vi "Create_filter_points.vi"(1 "Non-Blank Rows":bool[](array[boolean]), 5 "Precision":string, 6 "Channel to Filter On":i32, 7 "Tolerance":dbl=1.0 format="%.2f", 8 "Index":i32, 9 "Filter Bins 1":i32[](array[numeric]), 10 "Ch Values In":string[][](array[string])) -> (0 "Unchanged?":bool, 2 "Accept array":bool[][](array[boolean]), 3 "Filter Bins Out":i32[](array[numeric]), 4 "Bin Names":string[](array[string]))   [LabVIEW 2014]
uses:
  Results_plotter_Global.vi
panel:
  in  "Filter Info":T1={"Filter Bins"=[], "Channel to Filter On"=0, "Bin Matches"=[], "Number of Rows"=0, "Bin Names"=[], "Tolerance"=1.0, "Indicies for all bins"=[]} {"Tolerance" format="%.2f"}
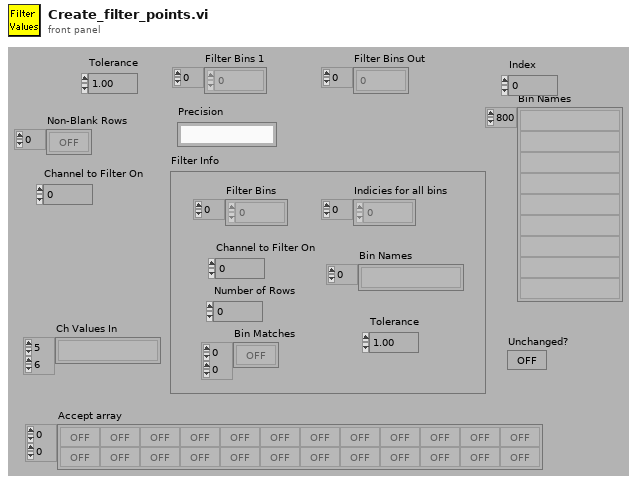
[diagram p1: front panel]
types:
  T1 = cluster{"Filter Bins":i32[], "Channel to Filter On":i32, "Bin Matches":bool[][], "Number of Rows":i32, "Bin Names":string[], "Tolerance":dbl, "Indicies for all bins":i32[]}
  T2 = cluster{"Filter Bins":i32[], "Channel to Filter On":i32, "Bin Matches":bool[][], "Number of Rows":i32, "Bin Names":string[], "Tolerance":dbl, "Indicies for all bins":i32[]}[]
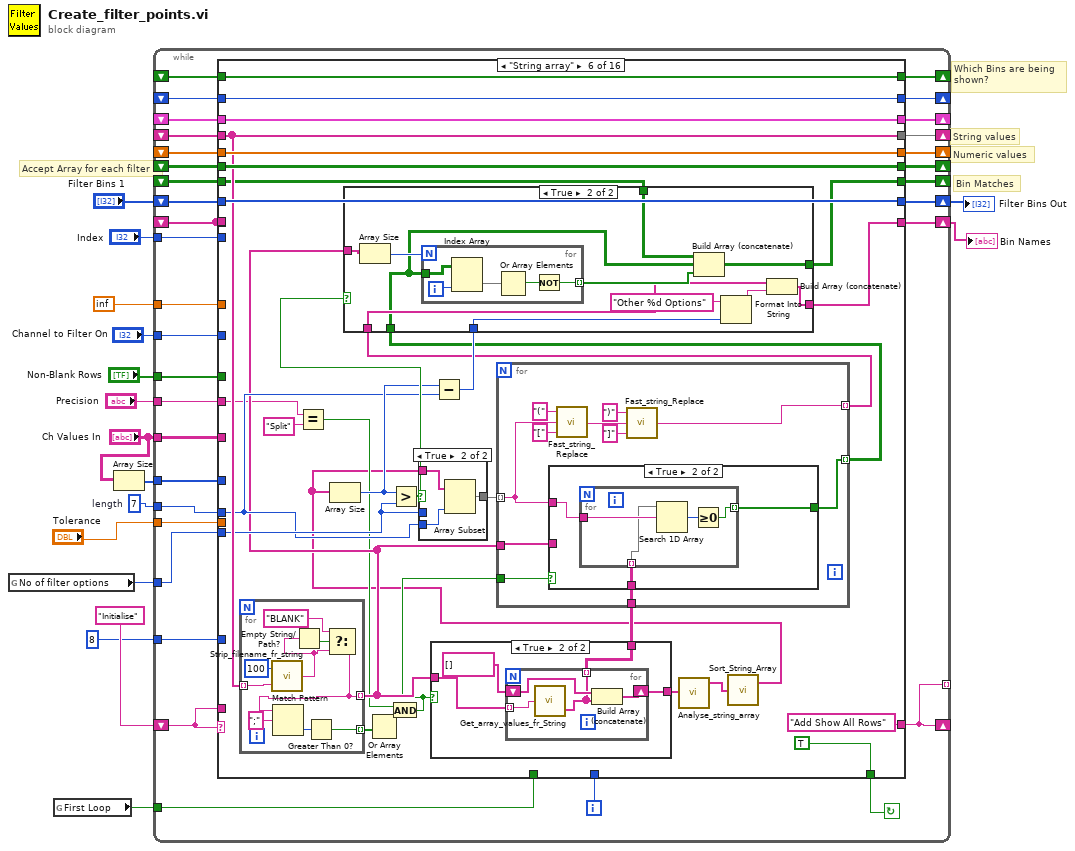
[diagram p0: block diagram]
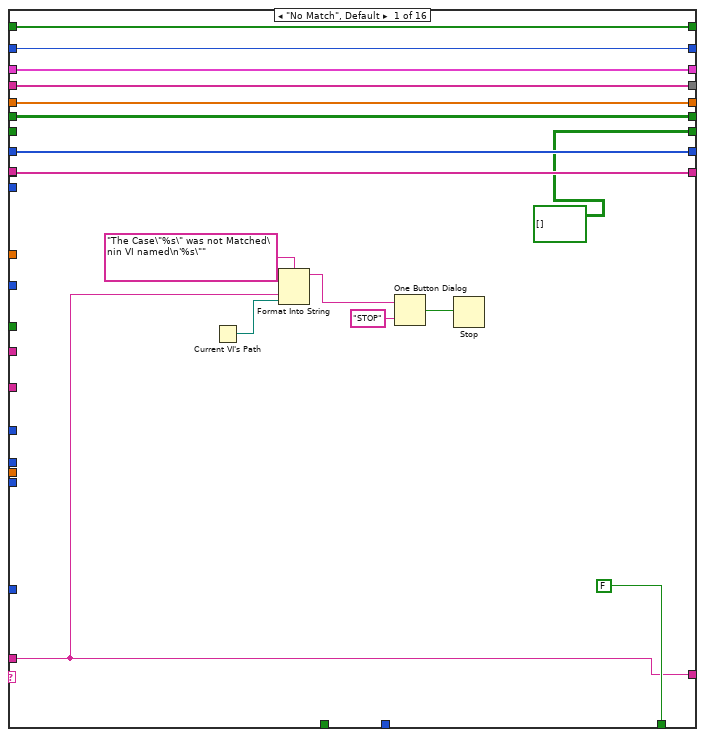
[diagram p2: hidden frame]
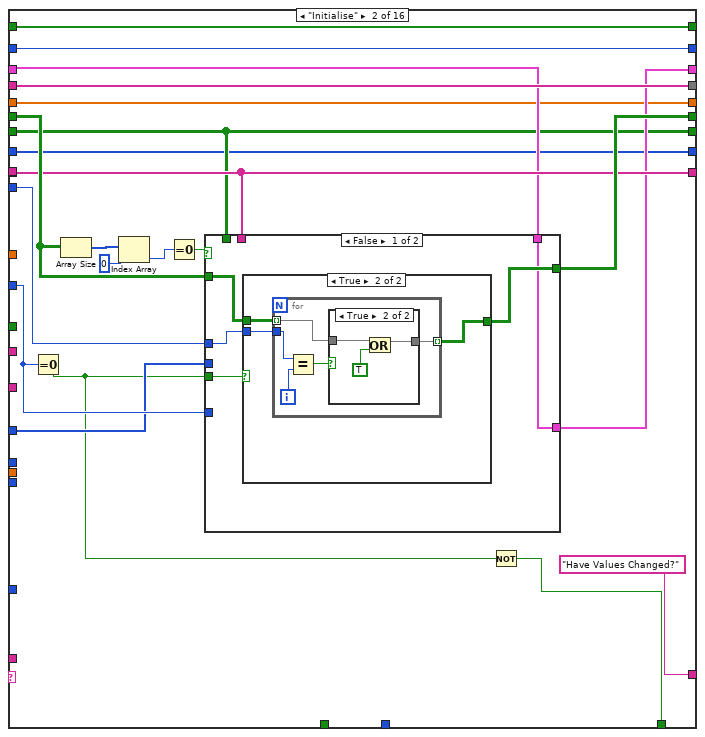
[diagram p3: hidden frame]
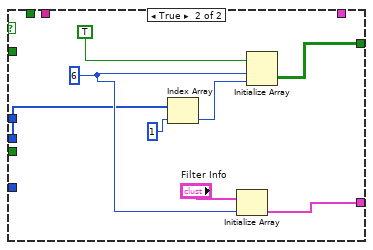
[diagram p6: hidden frame]
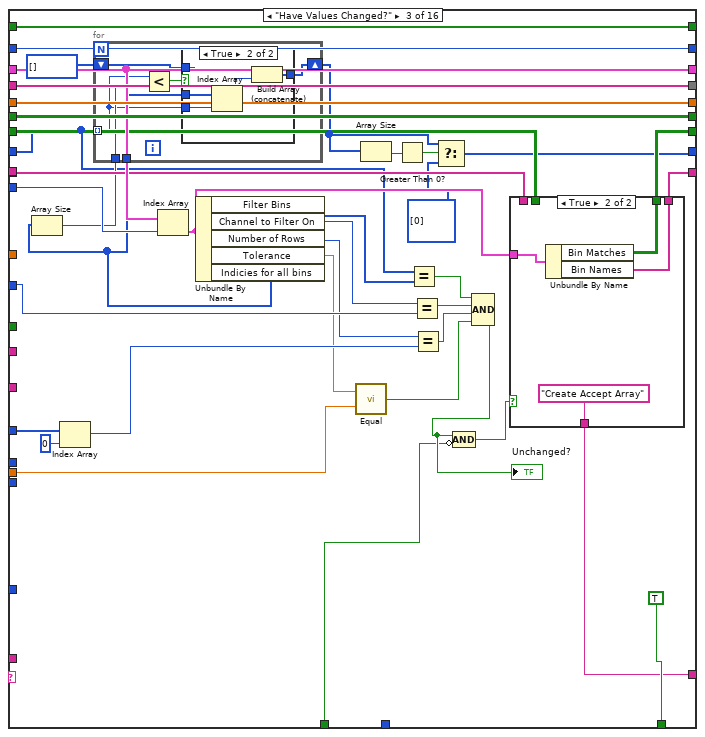
[diagram p7: hidden frame]
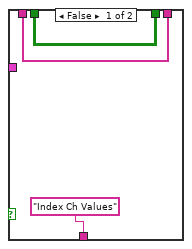
[diagram p9: hidden frame]
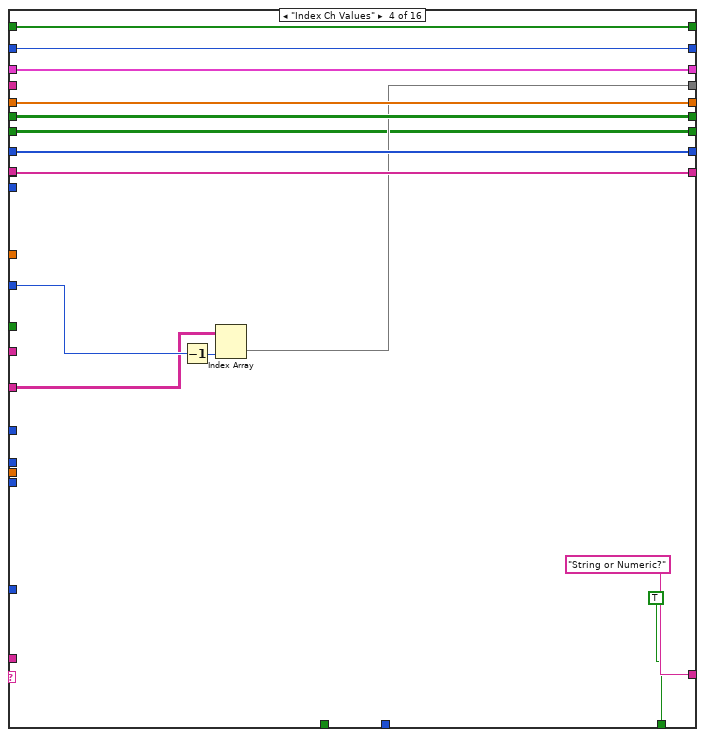
[diagram p10: hidden frame]
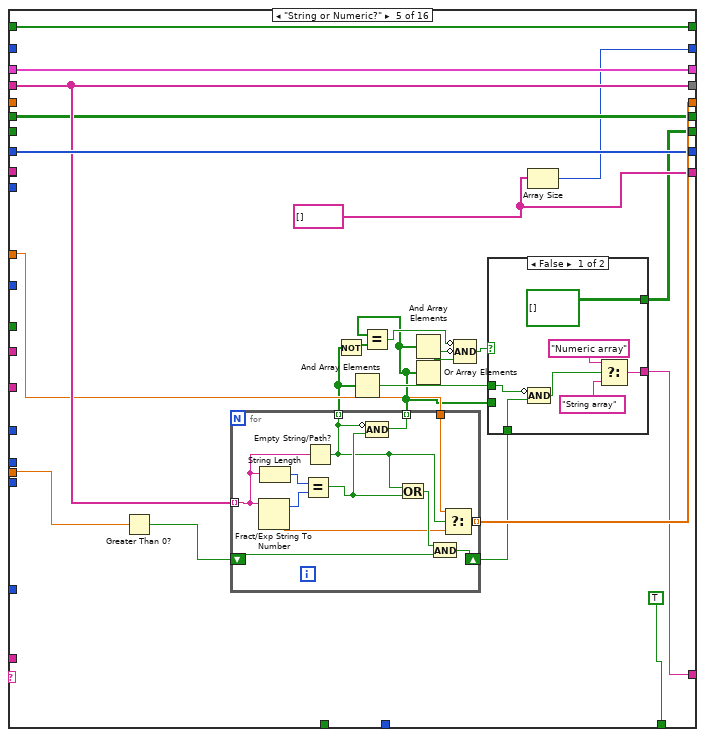
[diagram p11: hidden frame]
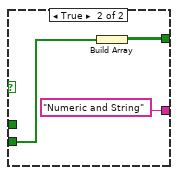
[diagram p12: hidden frame]
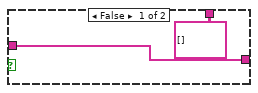
[diagram p13: hidden frame]
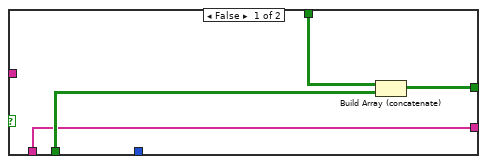
[diagram p14: hidden frame]
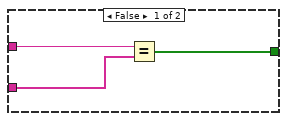
[diagram p16: hidden frame]
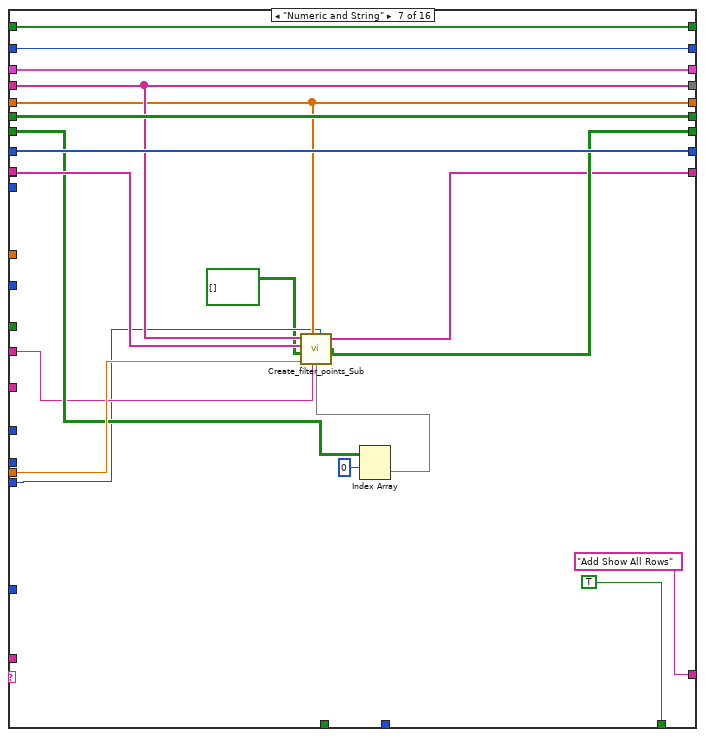
[diagram p17: hidden frame]
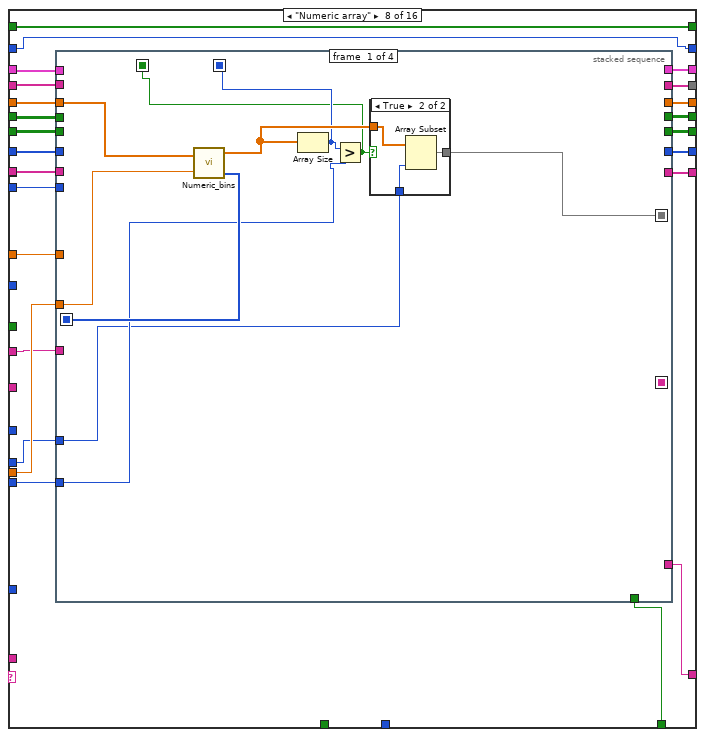
[diagram p18: hidden frame]
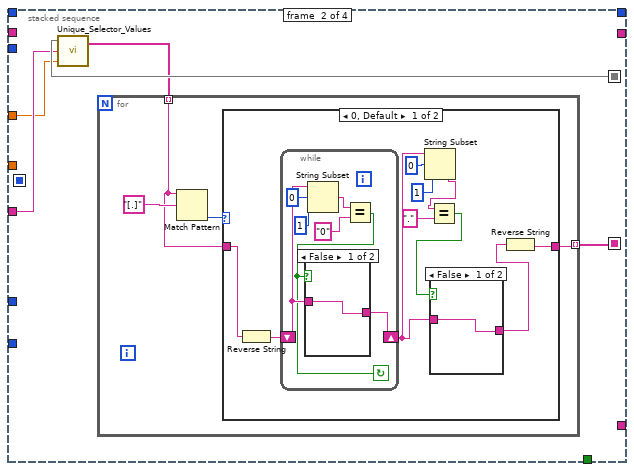
[diagram p20: hidden frame]
diagram:
  w5 = 7  # length
  # "Which Bins are being\nshown?"
  # "Accept Array for each filter"
  # "String values"
  # "Bin Matches"
  # "Numeric values"
  n1 = global read "Results_plotter_Global.vi" "No of filter options"() -> (w6:i32)
  n2 = global read "Results_plotter_Global.vi" "First Loop"() -> (w9:bool)
  n3 = Array Size(array="Ch Values In") -> (size(s)=w11:i32[])
  n4 = while {
    tunnel: "Non-Blank Rows" -> [w30]
    tunnel: w11 -> [w32]
    tunnel: "Channel to Filter On" -> [w34]
    shift-left: _ -> [w36]
    shift-right: [w35] -> _
    shift-left: _ -> [w37]
    shift-right: [w33] -> _
    shift-left: "Filter Bins 1" -> [w39]
    shift-right: [w38] -> w3
    tunnel: "Index" -> [w41]
    shift-left: _ -> [w40]
    shift-right: [w42] -> w14
    shift-left: _ -> [w27]
    shift-right: [w24] -> _
    shift-left: _ -> [w46]
    shift-right: [w45] -> _
    shift-left: _ -> [w43]
    shift-right: [w48] -> _
    shift-left: "Initialise" -> [w44]
    shift-right: [w17] -> _
    tunnel: inf -> [w49]
    tunnel: "Ch Values In" -> [w50]
    tunnel: w9 -> [w29]
    tunnel: "Tolerance" -> [w28]
    shift-right: [w26] -> _
    shift-left: _ -> [w25]
    tunnel: "Precision" -> [w23]
    shift-right: [w22] -> _
    shift-left: _ -> [w21]
    tunnel: w6 -> [w20]
    tunnel: w5 -> [w19]
    tunnel: 8 ("y") -> [w18]
    tunnel: [w17] -> _ mode=indexing
    i -> [w31]
    stop <- w47 continue-if-true
    n5 = case shown="\"String array\"" w44 {
      tunnel: w50 -> [_ _ _ w175 _ _ _ _ _ _ _ _ _ _ _ _]
      tunnel: w49 -> [_ _ _ _ w201 _ _ w358 _ _ _ _ _ _ _ _]
      tunnel: [w65 w73 w151 w183 w208 w260 w332 w365 w482 w500 w520 w562 w614 w632 w659 w698] -> w48
      tunnel: [w55 "Have Values Changed?" w135 "String or Numeric?" w192 "Add Show All Rows" "Add Show All Rows" w367 w465 "Create Accept Array" "Add Number of hits" "Relocate Selector?" w603 "Stop invalid selections" "Update shift Register" "End"] -> w17
      tunnel: [FALSE w76 TRUE TRUE TRUE TRUE TRUE w368 TRUE TRUE TRUE TRUE TRUE TRUE TRUE FALSE] -> w47
      tunnel: w46 -> [w64 w83 w150 w182 w202 w257 w341 w363 w481 w499 w515 w559 w612 w631 w658 w697]
      tunnel: [w64 w84 w150 w182 w202 w257 w341 w362 w481 w499 w514 w559 w612 w631 w658 w697] -> w45
      tunnel: w44 -> [w55 _ _ _ _ _ _ _ _ _ _ _ _ _ _ _]
      tunnel: w43 -> [w65 w73 w151 w183 _ w260 w332 w364 w482 w500 w520 w562 w614 w632 w659 w698]
      tunnel: [w63 w79 w134 w180 w188 w247 w333 w366 w469 w487 w518 w557 w611 w629 w656 w677] -> w42
      tunnel: w41 -> [_ w82 w148 _ _ _ _ w357 _ _ w517 w563 w601 w628 _ w695]
      tunnel: w27 -> [_ w74 w136 w174 _ w250 w335 w360 w475 w492 w507 w551 w613 w624 w654 w688]
      tunnel: w40 -> [w63 w79 w133 w180 _ _ w336 w351 w474 w488 w518 w554 w611 w629 w656 w680]
      tunnel: w40 -> [_ _ _ _ _ _ _ _ _ _ _ _ _ _ _ _]
      tunnel: w39 -> [w54 w72 w114 w181 w206 w256 w340 w359 w485 w503 w512 w566 w616 w622 w652 w675]
      tunnel: [w54 w72 w115 w181 w206 w256 w340 w352 w485 w503 w512 w566 w616 w617 w648 w674] -> w38
      tunnel: w37 -> [w62 w81 w149 _ w204 w254 w339 w356 w483 w501 w521 w564 w615 w630 w657 w696]
      tunnel: w36 -> [w61 w77 w147 w179 w205 w258 w342 w354 w484 w502 w522 w565 w609 w620 w651 w694]
      tunnel: [w61 w78 w147 w179 w205 w258 w342 w353 w484 w502 w522 w565 w609 w620 w651 w693] -> w35
      tunnel: w34 -> [_ w80 w146 w177 _ _ _ _ _ _ _ _ _ _ _ w687]
      tunnel: [w62 w81 w149 w176 w204 w254 w339 w355 w483 w501 w521 w564 w615 w630 w657 w696] -> w33
      tunnel: [bool[][] [] w74 w123 w174 w187 w248 w334 w361 w464 w491 w507 w551 w613 w624 w654 w688] -> w24
      tunnel: w32 -> [_ w71 w145 _ _ _ _ _ w479 _ _ _ _ _ _ w692]
      tunnel: w31 -> [_ _ _ _ _ _ _ _ _ _ _ _ _ _ _ _]
      tunnel: w30 -> [_ _ _ _ _ _ _ _ _ _ w511 w561 _ _ _ _]
      tunnel: w29 -> [_ _ w127 _ _ _ _ _ _ _ _ _ _ _ _ _]
      tunnel: w28 -> [_ _ w126 _ w191 _ w338 w350 _ _ _ _ _ _ _ w683]
      tunnel: [w53 w68 w125 w173 w190 w255 w331 w345 w471 w496 w509 w558 w600 w619 w650 w682] -> w26
      tunnel: w25 -> [w53 w68 w125 w173 _ w255 w331 w345 w471 w496 w509 w558 w600 w619 w650 w682]
      tunnel: w23 -> [_ _ _ _ _ w236 w330 w349 _ _ _ _ _ _ _ _]
      tunnel: [w51 w67 w124 w172 w189 w253 w329 w348 w470 w486 w508 w556 w599 w618 w649 w681] -> w22
      tunnel: w21 -> [w51 w67 w124 w172 w189 w253 w329 w348 w470 w486 w508 _ w599 w618 w649 w681]
      tunnel: w20 -> [_ _ _ _ _ w251 w328 w347 _ _ _ w543 _ _ _ _]
      tunnel: w19 -> [_ _ _ _ _ w245 _ w346 _ _ _ _ _ _ _ _]
      tunnel: w18 -> [_ _ _ _ _ _ _ _ w462 _ _ w545 _ _ _ _]
      frame "No Match", Default {
        n6 = Current VI's Path() -> (path=w56:path)
        n7 = Format Into String(format string="The Case\"%s\" was not Matched\nin VI named\n'%s\"" ("Format String"), w55, w56) -> (resulting string=w59:string)  [unwired: 2 in, 1 out]
        n8 = One Button Dialog(message=w59, button name ("OK")="STOP") -> (true=w57:bool)
        n9 = Stop(stop? (T)=w57) -> ()
      }
      frame "Initialise" {
        n10 = Equal To 0?(x=w80) -> (x = 0?=w70:bool)
        n11 = Array Size(array=w83) -> (size(s)=w87:i32[])
        n12 = Index Array(array=w87, index=0 ("Index")) -> (element=w85:i32)
        n13 = Equal To 0?(x=w85) -> (x = 0?=w69:bool)
        n14 = case shown="False" w69 {
          tunnel: [w92 w112] -> w84
          tunnel: w83 -> [w91 _]
          tunnel: w82 -> [w90 _]
          tunnel: w70 -> [w89 _]
          tunnel: w80 -> [_ _]
          tunnel: w79 -> [_ _]
          tunnel: [w88 w110] -> w78
          tunnel: w77 -> [w88 _]
          tunnel: w74 -> [_ _]
          tunnel: w71 -> [_ w107]
          frame False {
            n15 = case shown="True" w89 {
              tunnel: [w93 w95] -> w92
              tunnel: w91 -> [w93 w94]
              tunnel: w90 -> [_ w96]
              frame False {
              }
              frame True {
                n16 = for {
                  tunnel: w96 -> [w101]
                  tunnel: [w98] -> w95 mode=indexing
                  tunnel: w94 -> [w97] mode=indexing
                  i -> [w100]
                  n17 = Equal?(x=w101, y=w100) -> (x = y?=w99:bool)
                  n18 = case shown="True" w99 {
                    tunnel: [w102 w103] -> w98
                    tunnel: w97 -> [w102 w104]
                    frame False {
                    }
                    frame True {
                      n19 = Or(x=w104, y=TRUE) -> (x .or. y?=w103:bool[])
                    }
                  }
                }
              }
            }
          }
          frame True {
            w111 = 6 ("Dimension Size")
            n20 = Index Array(array=w107, index=1 ("Index")) -> (element=w108:i32)
            n21 = Initialize Array("Filter Info", w111) -> (w110:T2)
            n22 = Initialize Array(TRUE, w111, w108) -> (w112:bool[][])
          }
        }
        n23 = Not(x=w70) -> (.not. x?=w76:bool)
      }
      frame "Have Values Changed?" {
        n24 = Index Array(array=w145, index=0 ("Index")) -> (element=w141:i32)
        n25 = Index Array(array=w147, index=w148) -> (element=w137:T1)
        n26 = Unbundle By Name(w137) -> ("Filter Bins"=w132:i32[], "Channel to Filter On"=w143:i32, "Number of Rows"=w142:i32, "Tolerance"=w129:dbl, "Indicies for all bins"=w122:i32[])
        n27 = Array Size(array=w122) -> (size(s)=w121:i32)
        n28 = for {
          tunnel: w114 -> [w156] mode=indexing
          tunnel: w122 -> [w158]
          tunnel: w121 -> [w157]
          shift-right: [w154] -> w117
          shift-left: i32[] [] -> [w153]
          n29 = Less?(x=w156, y=w157) -> (x < y?=w155:bool)
          n30 = case shown="True" w155 {
            tunnel: w158 -> [_ w164]
            tunnel: w156 -> [_ w163]
            tunnel: [w159 w161] -> w154
            tunnel: w153 -> [w159 w160]
            frame False {
            }
            frame True {
              n31 = Index Array(array=w164, index=w163) -> (element=w162:i32)
              n32 = Build Array (concatenate)(w160, w162) -> (w161:i32[])
            }
          }
        }
        n33 = call "Equal.vi"("Input2"=w126, "Input1"=w129) -> ("Equal?"=w128:bool)
        n34 = Array Size(array=w117) -> (size(s)=w119:i32)
        n35 = Greater Than 0?(x=w119) -> (x > 0?=w118:bool)
        n36 = Equal?(x=w114, y=w132) -> (x = y?=w140:bool)
        n37 = Equal?(x=w143, y=w146) -> (x = y?=w139:bool)
        n38 = Equal?(x=w142, y=w141) -> (x = y?=w138:bool)
        n39 = Select(t=w117, s=w118, f=i32[] [0]) -> (s? t:f=w115:i32[])
        n40 = Compound Arithmetic op=AND(w140, w139, w138, w128) -> (w130:bool)
        "Unchanged?" <- w130
        n41 = Compound Arithmetic op=AND(w130, invert w127) -> (w131:bool)
        n42 = case shown="True" w131 {
          tunnel: w137 -> [_ w171]
          tunnel: [w165 w169] -> w123
          tunnel: w136 -> [w165 _]
          tunnel: ["Index Ch Values" "Create Accept Array"] -> w135
          tunnel: [w166 w170] -> w134
          tunnel: w133 -> [w166 _]
          frame False {
          }
          frame True {
            n43 = Unbundle By Name(w171) -> ("Bin Matches"=w169:bool[][], "Bin Names"=w170:string[])
          }
        }
      }
      frame "Index Ch Values" {
        n44 = Decrement(x=w177) -> (x-1=w178:i32)
        n45 = Index Array(array=w175, index (col)=w178) -> (element=w176:string[])  [unwired: 1 in]
      }
      frame "String or Numeric?" {
        w188 = string[] []
        n46 = Greater Than 0?(x=w191) -> (x > 0?=w207:bool)
        n47 = for {
          tunnel: w204 -> [w223] mode=indexing
          shift-right: [w228] -> w193
          shift-left: w207 -> [w229]
          tunnel: [w227] -> w208 mode=indexing
          tunnel: [w221] -> w196 mode=indexing
          tunnel: w201 -> [w220]
          tunnel: [w219] -> w186 mode=indexing
          n48 = Fract/Exp String To Number(string=w223) -> (offset past number=w225:i32, number=w226:dbl)  [unwired: 3 out]
          n49 = String Length(string=w223) -> (length=w224:i32)
          n50 = Equal?(x=w224, y=w225) -> (x = y?=w222:bool)
          n51 = Empty String/Path?(string/path=w223) -> (empty?=w221:bool)
          n52 = Compound Arithmetic op=AND(invert w221, w222) -> (w219:bool)
          n53 = Or(x=w221, y=w222) -> (x .or. y?=w230:bool)
          n54 = And(x=w230, y=w229) -> (x .and. y?=w228:bool)
          n55 = Select(t=w220, s=w221, f=w226) -> (s? t:f=w227:dbl)
        }
        n56 = Not(x=w196) -> (.not. x?=w195:bool[])
        n57 = And Array Elements(Boolean array=w196) -> (logical AND=w194:bool)
        n58 = Equal?(x=w186, y=w195) -> (x = y?=w197:bool)
        n59 = And Array Elements(Boolean array=w186) -> (logical AND=w200:bool)
        n60 = Or Array Elements(Boolean array=w186) -> (logical OR=w199:bool)
        n61 = Compound Arithmetic op=AND(invert w197, invert w200, w199) -> (w198:bool)
        n62 = case shown="False" w198 {
          tunnel: w194 -> [w215 _]
          tunnel: w193 -> [w214 _]
          tunnel: [w210 "Numeric and String"] -> w192
          tunnel: [bool[][] [] w216] -> w187
          tunnel: w186 -> [_ w217]
          frame False {
            n63 = Compound Arithmetic op=AND(invert w215, w214) -> (w211:bool)
            n64 = Select(t="Numeric array", s=w211, f="String array") -> (s? t:f=w210:string)
          }
          frame True {
            n65 = Build Array(w217) -> (w216:bool[][])
          }
        }
        n66 = Array Size(array=w188) -> (size(s)=w190:i32)
      }
      frame "String array" {
        n67 = for {
          tunnel: w254 -> [w304] mode=indexing
          tunnel: [w296] -> w239 mode=indexing
          tunnel: [w300] -> w241 mode=indexing
          n68 = call "Strip_filename_fr_string.vi"("Input String"=w304, "y"=100) -> ("Output String"=w297:string)
          n69 = Empty String/Path?(string/path=w297) -> (empty?=w299:bool)
          n70 = Select(t="BLANK", s=w299, f=w297) -> (s? t:f=w296:string)
          n71 = Match Pattern(string=w296, regular expression=";") -> (offset past match=w301:i32)  [unwired: 4 out]
          n72 = Greater Than 0?(x=w301) -> (x > 0?=w300:bool)
        }
        n73 = Equal?(x=w236, y="Split") -> (x = y?=w234:bool)
        n74 = Or Array Elements(Boolean array=w241) -> (logical OR=w235:bool)
        n75 = And(x=w234, y=w235) -> (x .and. y?=w233:bool)
        n76 = case shown="True" w233 {
          tunnel: [w263 w266] -> w240
          tunnel: w239 -> [w263 w265]
          tunnel: [string[][] [] ("String array") w264] -> w238
          frame False {
          }
          frame True {
            n77 = for {
              shift-right: [w271] -> w266
              shift-left: string[] [] -> [w270]
              tunnel: w265 -> [w269] mode=indexing
              tunnel: [w268] -> w264 mode=indexing
              n78 = call "Get_array_values_fr_String.vi"("String Value"=w269) -> ("String array"=w268:string[])  [unwired: 1 out]
              n79 = Build Array (concatenate)(w270, w268) -> (w271:string[])
            }
          }
        }
        n80 = call "Analyse_string_array.vi"("String array"=w240) -> ("Unique strings"=w232:string[])  [unwired: 2 out]
        n81 = call "Sort_String_Array.vi"("Unsorted String"=w232) -> ("Sorted String"=w231:string[])  [unwired: 1 out]
        n82 = Array Size(array=w231) -> (size(s)=w246:i32)
        n83 = Greater?(x=w246, y=w251) -> (0:w249:bool)
        n84 = case shown="True" w249 {
          tunnel: w231 -> [w292 w295]
          tunnel: w251 -> [_ _]
          tunnel: [w292 w294] -> w252
          tunnel: w245 -> [_ w293]
          frame False {
          }
          frame True {
            n85 = Array Subset(array=w295, length=w293) -> (w294:string[])  [unwired: 1 in]
          }
        }
        n86 = Subtract(x=w246, y=w245) -> (x-y=w244:i32)
        n87 = for {
          tunnel: w239 -> [w310]
          tunnel: w252 -> [w309] mode=indexing
          tunnel: [w305] -> w243 mode=indexing
          tunnel: [w308] -> w242 mode=indexing
          tunnel: w233 -> [w307]
          tunnel: w238 -> [w306]
          n88 = case shown="True" w307 {
            tunnel: w310 -> [w318 _]
            tunnel: w309 -> [w317 w321]
            tunnel: [w316 w320] -> w308
            tunnel: w306 -> [_ w319]
            frame False {
              n89 = Equal?(x=w317, y=w318) -> (x = y?=w316:bool[])
            }
            frame True {
              n90 = for {
                tunnel: w321 -> [w325]
                tunnel: [w323] -> w320 mode=indexing
                tunnel: w319 -> [w322] mode=indexing
                n91 = Search 1D Array(1D array=w322, element=w325) -> (index of element=w324:i32)  [unwired: 1 out]
                n92 = Greater Or Equal To 0?(x=w324) -> (x >= 0?=w323:bool)
              }
            }
          }
          n93 = call "Fast_string_Replace.vi"("Replace match with:"="[", "Input String"=w309, "regular expression"="(") -> ("Output String"=w311:string)  [unwired: 2 out]
          n94 = call "Fast_string_Replace.vi"("Replace match with:"="]", "Input String"=w311, "regular expression"=")") -> ("Output String"=w305:string)  [unwired: 2 out]
        }
        n95 = case shown="True" w249 {
          tunnel: w243 -> [w273 w283]
          tunnel: w250 -> [w275 w286]
          tunnel: w242 -> [w274 w276]
          tunnel: [w272 w284] -> w248
          tunnel: [w273 w282] -> w247
          tunnel: w239 -> [_ w281]
          tunnel: w244 -> [_ w279]
          frame False {
            n96 = Build Array (concatenate)(w275, w274) -> (w272:bool[][])
          }
          frame True {
            n97 = Array Size(array=w281) -> (size(s)=w280:i32)
            n98 = for {
              N: w280 -> [_]
              tunnel: w276 -> [w291]
              tunnel: [w287] -> w285 mode=indexing
              i -> [w290]
              n99 = Index Array(array=w291, index (col)=w290) -> (element=w289:bool[])  [unwired: 1 in]
              n100 = Or Array Elements(Boolean array=w289) -> (logical OR=w288:bool)
              n101 = Not(x=w288) -> (.not. x?=w287:bool)
            }
            n102 = Build Array (concatenate)(w286, w276, w285) -> (w284:bool[][])
            n103 = Format Into String(format string="Other %d Options", w279) -> (resulting string=w277:string)  [unwired: 2 in, 1 out]
            n104 = Build Array (concatenate)(w283, w277) -> (w282:string[])
          }
        }
      }
      frame "Numeric and String" {
        n105 = Index Array(array=w335, index (row)=0) -> (element=w337:bool[])  [unwired: 1 in]
        n106 = call "Create_filter_points_Sub.vi"("Numeric Value?"=w337, "No of filter options"=w328, "Precision"=w330, "Tolerance"=w338, "Bin Matches in"=bool[][] [] ("Bin Matches"), "Numeric Array"=w332, "Bin Names In"=w336, "String Array"=w339) -> ("Bin Matches"=w334:bool[][], "Bin Names"=w333:string[])  [unwired: 1 out]
      }
      frame "Numeric array" {
        n107 = stacked-sequence {
          seq-local: [w369 _ _ _] -> [_ w386 w418 _]
          seq-local: [w375 _ _ _] -> [_ _ w430 _]
          seq-local: [_ w383 _ _] -> [_ _ w431 _]
          seq-local: [w371 _ _ _] -> [_ _ w429 _]
          seq-local: [w370 _ _ _] -> [_ _ w426 _]
          tunnel: w350 -> [w376 _ _ _]
          tunnel: [_ _ _ w457] -> w365
          tunnel: w364 -> [w377 _ _ w457]
          tunnel: w363 -> [_ _ _ w456]
          tunnel: [_ _ _ w456] -> w362
          tunnel: [_ _ w423 _] -> w361
          tunnel: w360 -> [_ _ w422 _]
          tunnel: w359 -> [_ _ _ w455]
          tunnel: [_ _ _ w455] -> w352
          tunnel: [_ _ _ TRUE] -> w368
          tunnel: [_ _ _ "Add Show All Rows"] -> w367
          tunnel: w358 -> [_ w382 _ _]
          tunnel: [_ _ w420 _] -> w366
          tunnel: w357 -> [_ _ _ _]
          tunnel: w356 -> [_ _ _ w459]
          tunnel: [_ _ _ w459] -> w355
          tunnel: w354 -> [_ _ _ w458]
          tunnel: [_ _ _ w458] -> w353
          tunnel: w351 -> [_ _ w419 _]
          tunnel: w349 -> [_ w385 _ _]
          tunnel: w347 -> [w373 _ _ _]
          tunnel: w346 -> [w372 _ w428 _]
          frame #0 {
            n108 = call "Numeric_bins.vi"("Values"=w377, "Tolerance"=w376) -> ("Bin Centres"=w374:dbl[], "Bin Index"=w375:i32[])  [unwired: 1 out]
            n109 = Array Size(array=w374) -> (size(s)=w371:i32)
            n110 = Greater?(x=w371, y=w373) -> (0:w370:bool)
            n111 = case shown="True" w370 {
              tunnel: w374 -> [w378 w381]
              tunnel: [w378 w380] -> w369
              tunnel: w372 -> [_ w379]
              frame False {
              }
              frame True {
                n112 = Array Subset(array=w381, length=w379) -> (w380:dbl[])  [unwired: 1 in]
              }
            }
          }
          frame #1 {
            n113 = call "Unique_Selector_Values.vi"("Number that means blank"=w382, "Precision"=w385, "Bin Centres"=w386) -> ("Bin Strings"=w384:string[])  [unwired: 1 out]
            n114 = for {
              tunnel: [w388] -> w383 mode=indexing
              tunnel: w384 -> [w387] mode=indexing
              n115 = Match Pattern(string=w387, regular expression="[.]") -> (offset past match=w389:i32)  [unwired: 4 out]
              n116 = case shown="0, Default" w389 {
                tunnel: [w398 w416] -> w388
                tunnel: w387 -> [w400 w416]
                frame 0, Default {
                  n117 = Reverse String(1:w400) -> (0:w399:string)
                  n118 = while {
                    shift-right: [w406] -> w393
                    shift-left: w399 -> [w407]
                    stop <- w405 continue-if-true
                    n119 = String Subset(string=w407, offset (0)=0, length (rest)=1 ("length (rest)")) -> (substring=w409:string)
                    n120 = Equal?(x=w409, y="0") -> (x = y?=w405:bool)
                    n121 = case shown="False" w405 {
                      tunnel: w407 -> [w412 w414]
                      tunnel: [w412 w413] -> w406
                      frame False {
                      }
                      frame True {
                        n122 = String Subset(string=w414, offset (0)=1) -> (substring=w413:string)  [unwired: 1 out]
                      }
                    }
                  }
                  n123 = String Subset(string=w393, offset (0)=0, length (rest)=1 ("length (rest)")) -> (substring=w395:string)
                  n124 = Equal?(x=w395, y=".") -> (x = y?=w392:bool)
                  n125 = case shown="False" w392 {
                    tunnel: w393 -> [w401 w403]
                    tunnel: [w401 w402] -> w391
                    frame False {
                    }
                    frame True {
                      n126 = String Subset(string=w403, offset (0)=1) -> (substring=w402:string)  [unwired: 1 out]
                    }
                  }
                  n127 = Reverse String(1:w391) -> (0:w398:string)
                }
                frame -1 {
                }
              }
            }
          }
          frame #2 {
            n128 = Array Size(array=w418) -> (size(s)=w417:i32)
            n129 = Subtract(x=w429, y=w428) -> (x-y=w427:i32)
            n130 = for {
              N: w417 -> [_]
              tunnel: w430 -> [w451]
              tunnel: [w450] -> w424 mode=indexing
              i -> [w449]
              n131 = for {
                tunnel: w451 -> [w454] mode=indexing
                tunnel: w449 -> [w453]
                tunnel: [w452] -> w450 mode=indexing
                n132 = Equal?(x=w453, y=w454) -> (x = y?=w452:bool)
              }
            }
            n133 = case shown="True" w426 {
              tunnel: w431 -> [w433 w441]
              tunnel: w424 -> [w432 w435]
              tunnel: [w432 w442] -> w425
              tunnel: [w433 w440] -> w421
              tunnel: w430 -> [_ w439]
              tunnel: w427 -> [_ w434]
              frame False {
              }
              frame True {
                n134 = Array Size(array=w439) -> (size(s)=w438:i32)
                n135 = for {
                  N: w438 -> [_]
                  tunnel: w435 -> [w448]
                  tunnel: [w444] -> w443 mode=indexing
                  i -> [w447]
                  n136 = Index Array(array=w448, index (col)=w447) -> (element=w446:bool[])  [unwired: 1 in]
                  n137 = Or Array Elements(Boolean array=w446) -> (logical OR=w445:bool)
                  n138 = Not(x=w445) -> (.not. x?=w444:bool)
                }
                n139 = Build Array (concatenate)(w435, w443) -> (w442:bool[][])
                n140 = Format Into String(format string="Other %d Options", w434) -> (resulting string=w436:string)  [unwired: 2 in, 1 out]
                n141 = Build Array (concatenate)(w441, w436) -> (w440:string[])
              }
            }
            n142 = Build Array (concatenate)(w419, w421) -> (w420:string[])
            n143 = Build Array (concatenate)(w422, w425) -> (w423:bool[][])
          }
          frame #3 {
          }
        }
      }
      frame "Add Show All Rows" {
        n144 = Index Array(array=w479, index=0 ("Index")) -> (element=w477:i32)
        n145 = Initialize Array(TRUE, w477) -> (w476:bool[])
        n146 = Build Array (concatenate)(w476, w475) -> (w464:bool[][])
        n147 = Build Array (concatenate)("Show All" ("Input Element"), w474) -> (w469:string[])
        n148 = Array Size(array=w469) -> (size(s)=w468:i32)
        n149 = Greater?(x=w468, y=w462) -> (0:w463:bool)
        n150 = Select(t="Create Accept Array", s=w463, f="Add NOT Selectors") -> (s? t:f=w465:string)
      }
      frame "Add NOT Selectors" {
        n151 = Increment(x=w496) -> (x+1=w495:i32)
        n152 = Array Subset(array=w492, index (row)=w495) -> (w494:bool[][])  [unwired: 3 in]
        n153 = Array Subset(array=w488, index=w495) -> (w490:string[])  [unwired: 1 in]
        n154 = Not(x=w494) -> (.not. x?=w493:bool[][])
        n155 = for {
          tunnel: w490 -> [w505] mode=indexing
          tunnel: [w504] -> w489 mode=indexing
          n156 = Concatenate Strings("NOT " ("string"), w505) -> (w504:string)
        }
        n157 = Build Array (concatenate)(w492, w493) -> (w491:bool[][])
        n158 = Build Array (concatenate)(w488, w489) -> (w487:string[])
      }
      frame "Create Accept Array" {
        n159 = for {
          tunnel: w512 -> [w538] mode=indexing
          tunnel: w507 -> [w537]
          shift-right: [w534] -> w516
          shift-left: _ -> [w535]
          tunnel: w511 -> [w533]
          tunnel: [w531] -> w510 mode=indexing
          i -> [w536]
          n160 = Index Array(array=w537, index (row)=w538) -> (element=w532:bool[])  [unwired: 1 in]
          n161 = And(x=w533, y=w532) -> (x .and. y?=w531:bool[])
          n162 = case shown="0" w536 {
            tunnel: w535 -> [_ w542]
            tunnel: [w539 w541] -> w534
            tunnel: w531 -> [w539 w540]
            frame 0 {
            }
            frame 1, Default {
              n163 = Or(x=w540, y=w542) -> (x .or. y?=w541:bool[])
            }
          }
        }
        "Accept array" <- w510
        n164 = for {
          tunnel: w517 -> [w527]
          tunnel: [w525] -> w514 mode=indexing
          tunnel: w515 -> [w524] mode=indexing
          tunnel: w516 -> [w523]
          i -> [w528]
          n165 = Equal?(x=w527, y=w528) -> (x = y?=w526:bool)
          n166 = case shown="False" w526 {
            tunnel: [w529 w530] -> w525
            tunnel: w524 -> [w529 _]
            tunnel: w523 -> [_ w530]
            frame False {
            }
            frame True {
            }
          }
        }
      }
      frame "Add Number of hits" {
        n167 = Array Size(array=w551) -> (size(s)=w550:i32[])
        n168 = Index Array(array=w550, index=0) -> (element=w548:i32)
        n169 = for {
          tunnel: w563 -> [w594]
          tunnel: w559 -> [w592] mode=indexing
          shift-right: [w590] -> w553
          shift-left: w561 -> [w591]
          i -> [w589]
          n170 = Equal?(x=w594, y=w589) -> (x = y?=w593:bool)
          n171 = case shown="False" w593 {
            tunnel: w592 -> [w597 _]
            tunnel: w591 -> [w596 w598]
            tunnel: [w595 w598] -> w590
            frame False {
              n172 = And(x=w597, y=w596) -> (x .and. y?=w595:bool[])
            }
            frame True {
            }
          }
        }
        n173 = Multiply(x=3, y=w545) -> (x*y=w546:i32)
        n174 = Less?(x=w548, y=w546) -> (x < y?=w547:bool)
        n175 = for {
          tunnel: w553 -> [w576]
          tunnel: w551 -> [w575] mode=indexing
          tunnel: w554 -> [w581] mode=indexing
          tunnel: [w580] -> w557 mode=indexing
          tunnel: [w572] -> w556 mode=indexing
          shift-right: [w573] -> _
          shift-left: 0 -> [w574]
          tunnel: w547 -> [w569]
          tunnel: w543 -> [w567]
          n176 = And(x=w576, y=w575) -> (x .and. y?=w577:bool[])
          n177 = Boolean To (0,1)(Boolean=w577) -> (0, 1=w578:i16[])
          n178 = To Long Integer(number=w578) -> (32bit integer=w568:i32[])
          n179 = Add Array Elements(numeric array=w568) -> (sum=w579:i32)
          n180 = Format Into String(format string=" (%d)" ("Format String"), initial string=w581, w579) -> (resulting string=w580:string)  [unwired: 1 in, 1 out]
          n181 = Greater Than 0?(x=w579) -> (x > 0?=w570:bool)
          n182 = Or(x=w570, y=w569) -> (x .or. y?=w571:bool)
          n183 = case shown="True" w571 {
            tunnel: w574 -> [w583 w587]
            tunnel: [w583 w588] -> w573
            tunnel: [FALSE w586] -> w572
            tunnel: w567 -> [_ w585]
            frame False {
            }
            frame True {
              n184 = Less?(x=w587, y=w585) -> (x < y?=w586:bool)
              n185 = Increment(x=w587) -> (x+1=w588:i32)
            }
          }
        }
      }
      frame "Relocate Selector?" {
        n186 = Index Array(array=w609, index=w601) -> (element=w610:T1)
        n187 = Unbundle By Name(w610) -> ("Bin Names"=w608:string[])
        n188 = Array Size(array=w608) -> (size(s)=w607:i32)
        n189 = Greater Than 0?(x=w607) -> (x > 0?=w605:bool)
        n190 = Select(t="Relocate Selector", s=w605, f="Stop invalid selections") -> (s? t:f=w603:string)
      }
      frame "Relocate Selector" {
        n191 = Index Array(array=w620, index=w628) -> (element=w625:T1)
        n192 = Unbundle By Name(w625) -> ("Bin Names"=w626:string[])
        n193 = for {
          tunnel: w629 -> [w635] mode=indexing
          tunnel: [w634] -> w623 mode=indexing
          n194 = Match Pattern(string=w635, regular expression=" (") -> (before substring=w634:string)  [unwired: 4 out]
        }
        n195 = for {
          tunnel: w622 -> [w637] mode=indexing
          tunnel: w626 -> [w643]
          tunnel: w623 -> [w641]
          shift-right: [w638] -> w617
          shift-left: i32[] [] -> [w639]
          n196 = Index Array(array=w643, index=w637) -> (element=w640:string)
          n197 = Search 1D Array(1D array=w641, element=w640) -> (index of element=w642:i32)  [unwired: 1 out]
          n198 = case shown="0, Default" w642 {
            tunnel: w642 -> [w644 _]
            tunnel: w639 -> [w646 w647]
            tunnel: [w645 w647] -> w638
            frame 0, Default {
              n199 = Build Array (concatenate)(w646, w644) -> (w645:i32[])
            }
            frame -1 {
            }
          }
        }
      }
      frame "Stop invalid selections" {
        n200 = Array Size(array=w652) -> (size(s)=w653:i32)
        n201 = case shown="2, Default" w653 {
          tunnel: [i32[] [0] w662 w663] -> w648
          tunnel: w652 -> [_ w662 w665]
          frame 0 {
          }
          frame 1 {
          }
          frame 2, Default {
            n202 = for {
              tunnel: w665 -> [w666] mode=indexing
              shift-right: [w667] -> w663
              shift-left: i32[] [] -> [w668]
              n203 = Equal To 0?(x=w666) -> (x = 0?=w669:bool)
              n204 = case shown="False" w669 {
                tunnel: w668 -> [w671 w673]
                tunnel: [w670 w673] -> w667
                tunnel: w666 -> [w672 _]
                frame False {
                  n205 = Build Array (concatenate)(w671, w672) -> (w670:i32[])
                }
                frame True {
                }
              }
            }
          }
        }
      }
      frame "Update shift Register" {
        n206 = Index Array(array=w694, index=w695) -> (element=w689:T1)
        n207 = Index Array(array=w692, index=0 ("Index")) -> (element=w685:i32)
        n208 = for {
          tunnel: w680 -> [w722] mode=indexing
          tunnel: [w721] -> w686 mode=indexing
          n209 = Match Pattern(string=w722, regular expression=" (") -> (before substring=w721:string)  [unwired: 4 out]
        }
        n210 = for {
          shift-right: [w706] -> w677
          shift-left: string[] [] -> [w709]
          tunnel: w681 -> [w712] mode=indexing
          shift-right: [w707] -> w676
          shift-left: i32[] [] -> [w708]
          tunnel: w680 -> [w710] mode=indexing
          i -> [w711]
          n211 = case shown="True" w712 {
            tunnel: w711 -> [_ w720]
            tunnel: w710 -> [_ w719]
            tunnel: w709 -> [w714 w718]
            tunnel: w708 -> [w713 w717]
            tunnel: [w713 w716] -> w707
            tunnel: [w714 w715] -> w706
            frame False {
            }
            frame True {
              n212 = Build Array (concatenate)(w718, w719) -> (w715:string[])
              n213 = Build Array (concatenate)(w717, w720) -> (w716:i32[])
            }
          }
        }
        n214 = for {
          tunnel: w676 -> [w705]
          tunnel: w675 -> [w704] mode=indexing
          tunnel: [w700] -> w674 mode=indexing
          n215 = Search 1D Array(1D array=w705, element=w704) -> (index of element=w701:i32)  [unwired: 1 out]
          n216 = In Range and Coerce(upper limit=65000, x=w701, lower limit=0) -> (coerced(x)=w700:i32)  [unwired: 1 out]
        }
        n217 = Bundle By Name(cluster=w689, "Bin Matches"=w688, "Channel to Filter On"=w687, "Bin Names"=w686, "Number of Rows"=w685, "Tolerance"=w683, "Filter Bins"=w674, "Indicies for all bins"=w676) -> (w684:T1)
        n218 = Replace Array Subset(array=w694, new element=w684, index=w695) -> (w693:T2)
      }
    }
  }
  "Bin Names" <- w14
  "Filter Bins Out" <- w3
